vi "ClearFaults.vi"(11 "Proccess in":refnum<class "Proccess.lvclass">) -> (3 "Proccess out":refnum<class "Proccess.lvclass">)   [LabVIEW 2019, in "Proccess.lvclass"]
uses:
  Proccess.lvclass
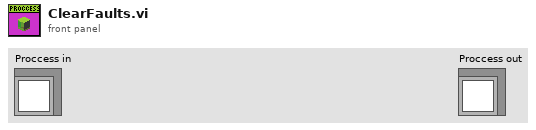
[diagram p1: front panel]
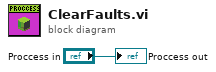
[diagram p0: block diagram]
diagram:
  "Proccess out" <- "Proccess in"
